vi "GetFunctionConfig.vi"(8 "error in (no error)":errorcluster, 11 "PmuTestFunctions In":refnum<class "PmuTestFunctions.lvclass">) -> (0 "error out":errorcluster, 2 "FunctionConfig":variant, 3 "PmuTestFunctions Out":refnum<class "PmuTestFunctions.lvclass">)   [LabVIEW 2018, in "Functions.lvlib" / "PmuTestFunctions.lvclass"]
uses:
  PmuTestFunctions.lvclass
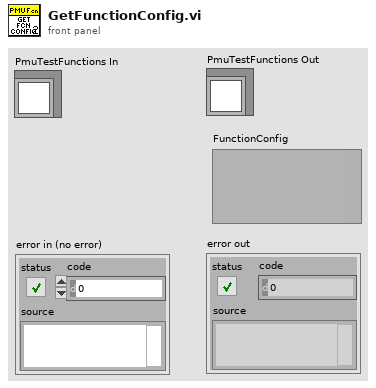
[diagram p1: front panel]
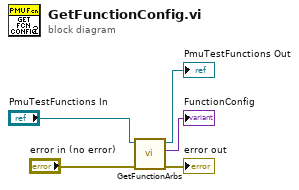
[diagram p0: block diagram]
diagram:
  n1 = call-dynamic "GetFunctionArbs.vi"("error in (no error)"="error in (no error)", "PmuTestFunctions in"="PmuTestFunctions In") -> ("error out"=→"error out":errorcluster, "Arbs"=→"FunctionConfig":variant, "PmuTestFunctions out"=→"PmuTestFunctions Out":refnum<class "PmuTestFunctions.lvclass">)  [unwired: 7 in]
